vi "MCcontrol_main.vi"() -> ()   [LabVIEW 2011]
uses:
  perHandlemonochromator.vi
  users/nicolas/PHySpec-SDK-1.0.0/Labview-example/libPhyspec/libPhyspec.lvlib
panel:
  in  "Refresh Button":bool
  in  "set Wavelength":dbl
  in  "stop":bool
  out "Current Wavelength":dbl
  out "error IO":errorcluster
  out "peHandle":u32
  out "MachineState":string="init"
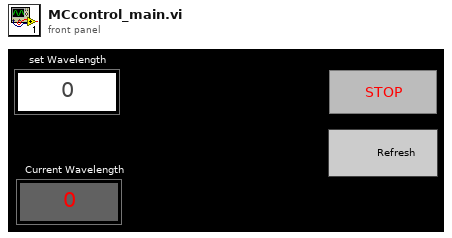
[diagram p1: front panel]
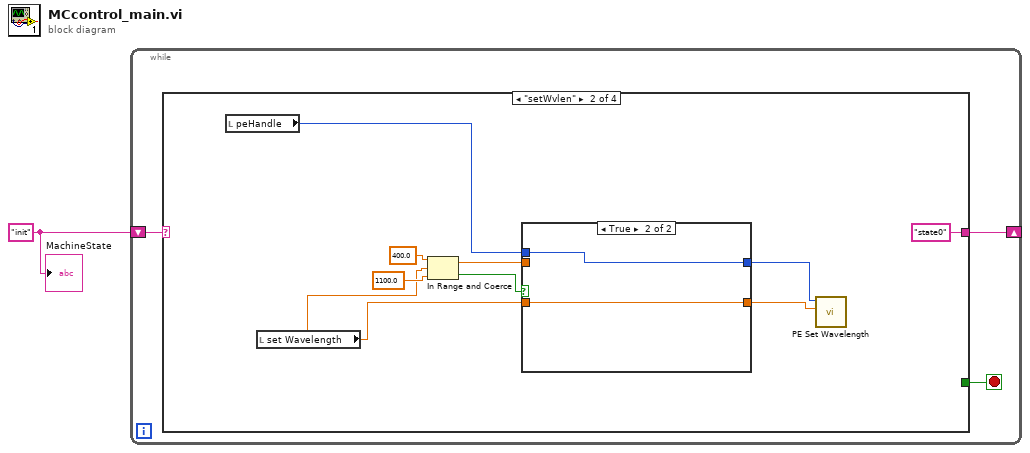
[diagram p0: block diagram]
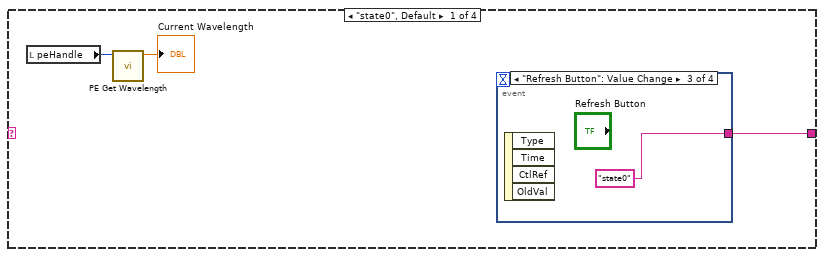
[diagram p2: hidden frame]
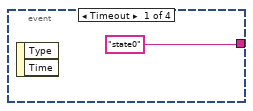
[diagram p3: hidden frame]
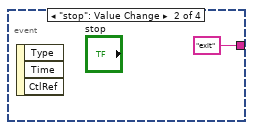
[diagram p4: hidden frame]
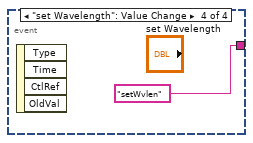
[diagram p5: hidden frame]
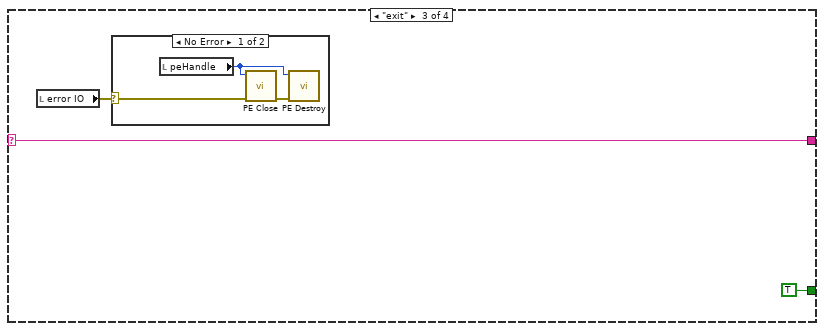
[diagram p7: hidden frame]
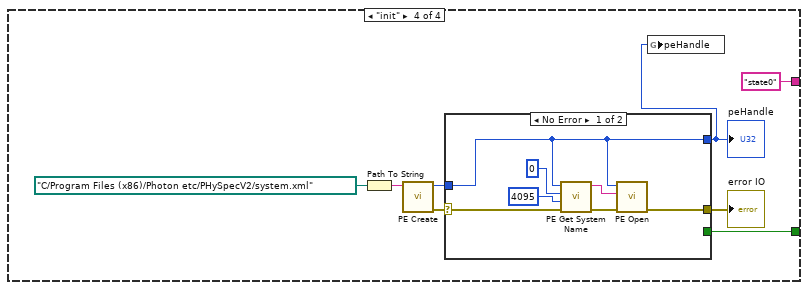
[diagram p9: hidden frame]
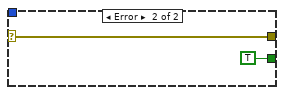
[diagram p10: hidden frame]
diagram:
  w1 = "init"
  n1 = while {
    shift-right: [w3] -> _
    shift-left: w1 -> [w4]
    stop <- w2 stop-if-true
    n2 = case shown="\"setWvlen\"" w4 {
      selector: w4 -> [_ _ w25 _]
      tunnel: [w5 "state0" w25 "state0"] -> w3
      tunnel: [_ _ TRUE w33] -> w2
      frame "state0", Default {
        n3 = local read "peHandle"() -> (w7:u32)
        n4 = call "PE Get Wavelength.vi"("peHandle"=w7) -> ("wavelength"=→"Current Wavelength":dbl)  [unwired: 8 in, 2 out]
        n5 = event shown="[2] \"Refresh Button\": Value Change" {
          selector: _ -> [_ _ _ _]
          dyn-events: _ -> [_ _ _ _]
          timeout: _ -> [_ _ _ _]
          tunnel: ["state0" "exit" "state0" "setWvlen"] -> w5
          event Timeout {
            n6 = event-data() -> ()  [unwired: 1 in, 2 out]
          }
          event "stop": Value Change {
            n7 = event-data() -> ()  [unwired: 1 in, 3 out]
          }
          event "Refresh Button": Value Change {
            n8 = event-data() -> ()  [unwired: 1 in, 4 out]
          }
          event "set Wavelength": Value Change {
            n9 = event-data() -> ()  [unwired: 1 in, 4 out]
          }
        }
      }
      frame "setWvlen" {
        n10 = local read "peHandle"() -> (w16:u32)
        n11 = local read "set Wavelength"() -> (w12:dbl)
        n12 = In Range and Coerce(upper limit=400.0, x=w12, lower limit=1100.0) -> (coerced(x)=w14:dbl, In Range?=w17:bool)
        n13 = case shown="True" w17 {
          tunnel: w16 -> [w22 w24]
          tunnel: [w22 w24] -> w15
          tunnel: w14 -> [w21 _]
          tunnel: [w21 w23] -> w13
          tunnel: w12 -> [_ w23]
          frame False {
          }
          frame True {
          }
        }
        n14 = call "PE Set Wavelength.vi"("wavelength"=w13, "peHandle"=w15) -> ()  [unwired: 8 in, 2 out]
      }
      frame "exit" {
        n15 = local read "error IO"() -> (w27:errorcluster)
        n16 = case shown="No Error" w27 {
          selector: w27 -> [w28 _]
          frame No Error {
            n17 = local read "peHandle"() -> (w29:u32)
            n18 = call "PE Close.vi"("error in (no error)"=w28, "peHandle"=w29) -> ("error out"=w30:errorcluster)  [unwired: 8 in, 1 out]
            n19 = call "PE Destroy.vi"("error in (no error)"=w30, "peHandle"=w29) -> ()  [unwired: 8 in, 2 out]
          }
          frame Error {
          }
        }
      }
      frame "init" {
        n20 = Path To String(path=path "C:/Program Files (x86)/Photon etc/PHySpecV2/system.xml" ("Configuration File")) -> (string=w36:string)
        n21 = call "PE Create.vi"("conffile"=w36) -> ("error out"=w38:errorcluster, "peHandle"=w37:u32)  [unwired: 8 in, 1 out]
        n22 = case shown="No Error" w38 {
          selector: w38 -> [w43 w47]
          tunnel: w37 -> [w40 _]
          tunnel: [w40 _] -> w31
          tunnel: [w39 w47] -> w32
          tunnel: [_ TRUE] -> w33
          frame No Error {
            n23 = call "PE Get System Name.vi"("error in (no error)"=w43, "size"=4095, "index"=0, "peHandle"=w40) -> ("error out"=w42:errorcluster, "name"=w41:string)  [unwired: 5 in, 1 out]
            n24 = call "PE Open.vi"("error in (no error)"=w42, "name"=w41, "peHandle"=w40) -> ("error out"=w39:errorcluster)  [unwired: 7 in, 1 out]
          }
          frame Error {
          }
        }
        "peHandle" <- w31
        "error IO" <- w32
        n25 = global write "perHandlemonochromator.vi" "peHandle"(w31) -> ()
      }
    }
  }
  "MachineState" <- w1
